vi "shutterOpen.vi"(6 "Delay between send and receive [ms]":i32=100, 8 "error in (no error)":errorcluster, 11 "Monochromator in":refnum<class "Monochromator.lvclass">) -> (0 "error out":errorcluster, 1 "ID":i32, 2 "results-JSON string":string, 3 "Monochromator out":refnum<class "Monochromator.lvclass">)   [LabVIEW 2023, in "Monochromator.lvclass"]
doc: "Activates the currently selected shutter solenoid.\n\nNote: The device must be configured for internal shutter mode. The shutter solenoid will not respond in External (Bypass) mode."
uses:
  Monochromator.lvclass
  Monochromator.lvclass/Monochromator.ctl
  7fe8abea-6ecd-46de-aa11-ce8637911b6a.vi
  GenericDevice/GenericDevice.lvclass
panel:
  # "Connector Pane"
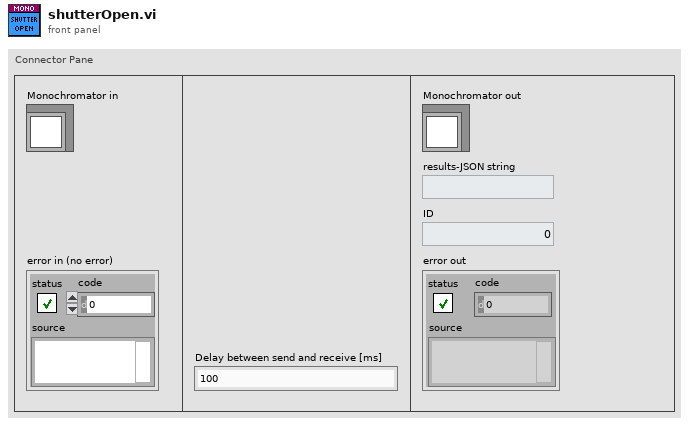
[diagram p1: front panel]
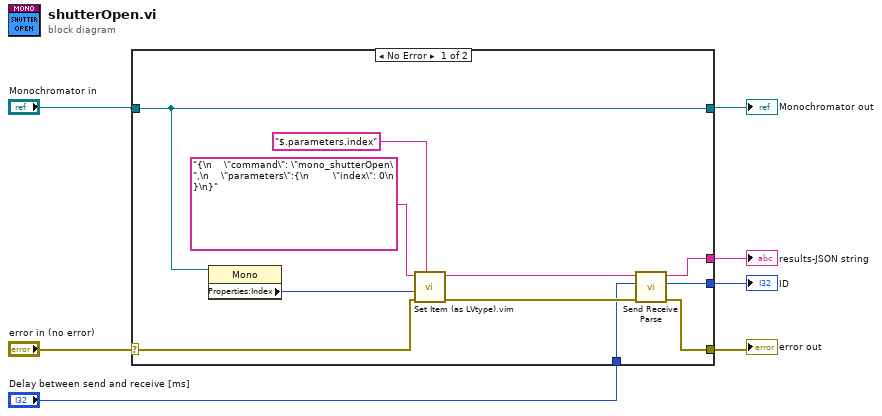
[diagram p0: block diagram]
diagram:
  n1 = case shown="No Error" "error in (no error)" {
    selector: "error in (no error)" -> [w14 w20]
    tunnel: [w11 w20] -> w4
    tunnel: [w16 w19] -> w6
    tunnel: "Monochromator in" -> [w16 w19]
    tunnel: [w13 _] -> w2
    tunnel: [w12 _] -> w3
    tunnel: "Delay between send and receive [ms]" -> [w8 _]
    frame No Error {
      n2 = property class="Mono"(reference=w16) -> ("Properties:Index"=w15:i32)  [unwired: 1 in, 2 out]
      n3 = call "Set Item (as LVtype).vim"("$Path or Item Name"="$.parameters.index", "error in (no error)"=w14, "Anything"=w15, "JSON"="{\n    \"command\": \"mono_shutterOpen\",\n    \"parameters\":{\n        \"index\": 0\n    }\n}") -> ("error out"=w9:errorcluster, "<JSON>"=w10:string)  [unwired: 4 in, 1 out]
      n4 = call "Send Receive Parse.vi"("error in"=w9, "Delay between send and receive [ms]"=w8, "<JSON>"=w10) -> ("error out"=w11:errorcluster, "ID"=w12:i32, "results-JSON string"=w13:string)  [unwired: 6 in]
    }
    frame Error {
    }
  }
  "error out" <- w4
  "Monochromator out" <- w6
  "ID" <- w3
  "results-JSON string" <- w2
